vi "MT_generate_signal2.vi"(9 "Amplitude":dbl, 10 "Frequency":dbl, 11 "Duration":dbl) -> (0 "error out":errorcluster, 2 "Signals out":dbl[][](array[numeric]), 3 "sample rate":dbl=1.0 format="%0.2f")   [LabVIEW 2019]
uses:
  <vilib>/Analysis/NI_AALPro.lvlib
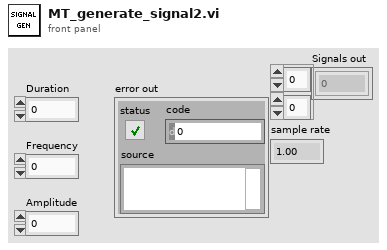
[diagram p1: front panel]
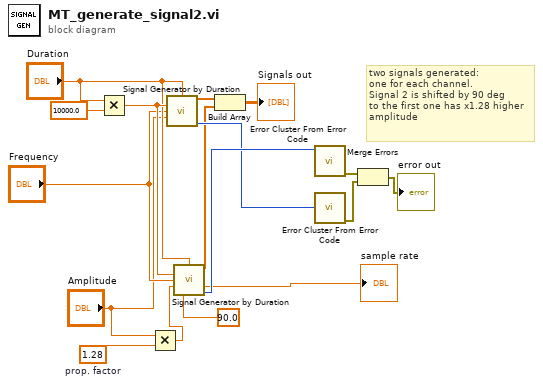
[diagram p0: block diagram]
diagram:
  w6 = 1.28  # prop. factor
  # "two signals generated:\none for each channel.\nSignal 2 is shifted by 90 deg\nto the first one has x1.28 higher\namplitude"
  n1 = Multiply(x="Duration", y=10000.0) -> (x*y=w14:dbl)
  n2 = Multiply(x="Amplitude", y=w6) -> (x*y=w4:dbl)
  n3 = call <vilib>:"Signal Generator by Duration.vi"("duration"="Duration", "# of samples"=w14, "frequency"="Frequency", "amplitude"="Amplitude") -> ("signal"=w9:dbl[], "error"=w10:i32)  [unwired: 8 in, 2 out]
  n4 = call <vilib>:"Signal Generator by Duration.vi"("duration"="Duration", "# of samples"=w14, "frequency"="Frequency", "amplitude"=w4, "phase in"=90.0) -> ("signal"=w8:dbl[], "sample rate"=→"sample rate":dbl, "error"=w11:i32)  [unwired: 7 in, 1 out]
  n5 = Build Array(w9, w8) -> (→"Signals out":dbl[][])
  n6 = call <vilib>:"Error Cluster From Error Code.vi"("error code (0)"=w11) -> ("error out"=w16:errorcluster)  [unwired: 8 in]
  n7 = call <vilib>:"Error Cluster From Error Code.vi"("error code (0)"=w10) -> ("error out"=w15:errorcluster)  [unwired: 8 in]
  n8 = Merge Errors(w16, w15) -> (→"error out":errorcluster)
